vi "Gyro.vi"(8 "ResetAngle":bool, 9 "GyroDevRef":T2 {"Sample Rate" min=0.25 max=100.0 step=0.25}) -> (3 "GyroData":T1)   [LabVIEW 2017]
uses:
  <vilib>/Rock Robotics/WPI/Gyro/WPI_GyroDevRef.ctl
  <vilib>/Rock Robotics/SystemInterfaces/AI/FPGA_AIChannel.ctl
  <vilib>/Rock Robotics/SystemInterfaces/spilib/spi_bus.ctl
  Gyro_TypeDef.ctl
panel:
  out "AngularRate":dbl
  out "Calibrated":bool
  out "Angle":dbl(knob) scale=0.0..360.0
  # "Analog"
  # "XRS"
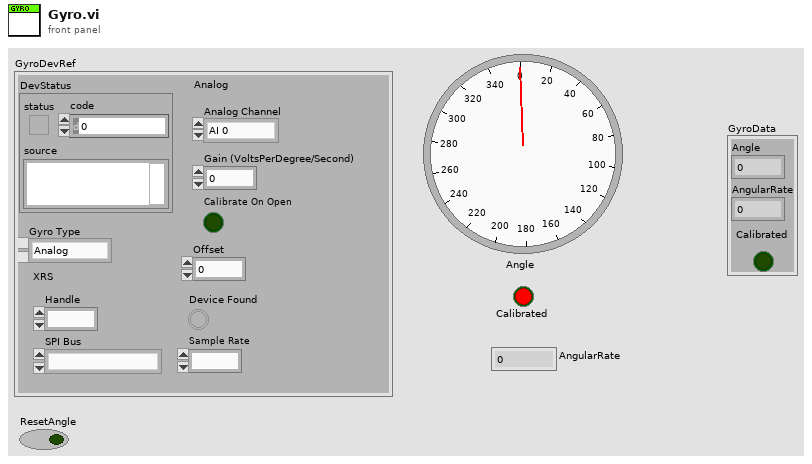
[diagram p1: front panel]
types:
  T1 = typedef "Gyro_TypeDef.ctl" = cluster{"Angle":dbl, "AngularRate":dbl, "Calibrated":bool}
  T2 = typedef "WPI_GyroDevRef.ctl" = cluster{"DevStatus":errorcluster, "Analog Channel":T3, "Gain (VoltsPerDegree/Second)":dbl, "Gyro Type":enum16{"Analog", "XRS450"}, "Handle":i32, "SPI Bus":T4, "Device Found":bool, "Sample Rate":dbl, "Calibrate On Open":bool, "Offset":dbl}
  T3 = typedef "FPGA_AIChannel.ctl" = enum8{"AI 0", "AI 1", "AI 2", "AI 3", "AI MXP 0", "AI MXP 1", "AI MXP 2", "AI MXP 3", "Invalid"}
  T4 = typedef "spi_bus.ctl" = enum16{"SPI On-Board, CS0", "SPI On-Board, CS1", "SPI On-Board, CS2", "SPI On-Board, CS3", "SPI MXP", "Invalid"}
  T5 = cluster{dbl, "Angular Rate":dbl, "Calibrated?":bool}
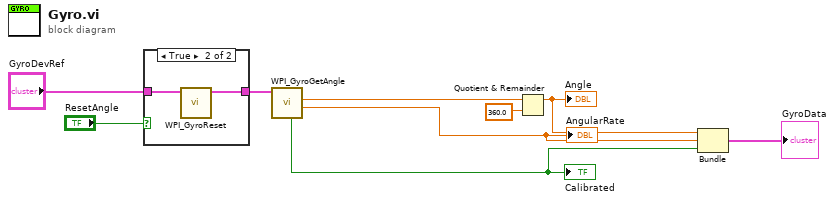
[diagram p0: block diagram]
diagram:
  n1 = case shown="True" "ResetAngle" {
    tunnel: "GyroDevRef" -> [w10 w12]
    tunnel: [w10 w11] -> w7
    frame False {
    }
    frame True {
      n2 = call <vilib>:"WPI_GyroReset.vi"("GyroDevRef"=w12) -> ("GyroDevRef"=w11:T2)  [unwired: 9 in, 1 out]
    }
  }
  n3 = call <vilib>:"WPI_GyroGetAngle.vi"("GyroDevRef"=w7) -> ("Angular Rate"=w3:dbl, "Angle"=w8:dbl, "Calibrated?"=w2:bool)  [unwired: 6 in, 2 out]
  "Calibrated" <- w2
  "AngularRate" <- w3
  n4 = Quotient & Remainder(x=w8, y=360.0) -> (x-y*floor(x/y)=w4:dbl)  [unwired: 1 out]
  "Angle" <- w4
  n5 = Bundle(w4, "Angular Rate"=w3, "Calibrated?"=w2) -> (→"GyroData":T5)  [unwired: 1 in]
